vi "MSScript_Transform_BooleanArray.vi"(8 "MinSize":u8=1, 9 "MaxSize":u8=1, 11 "Check_Str":string) -> (2 "Value Error?":bool, 3 "Value Output":bool[](array[boolean]))   [LabVIEW 2018, in "MSScript.lvclass"]
uses:
  MSScript.lvclass
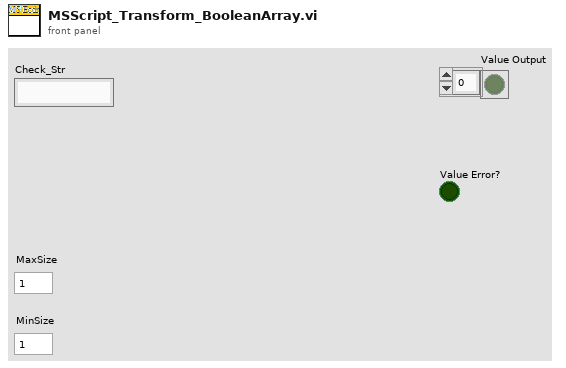
[diagram p1: front panel]
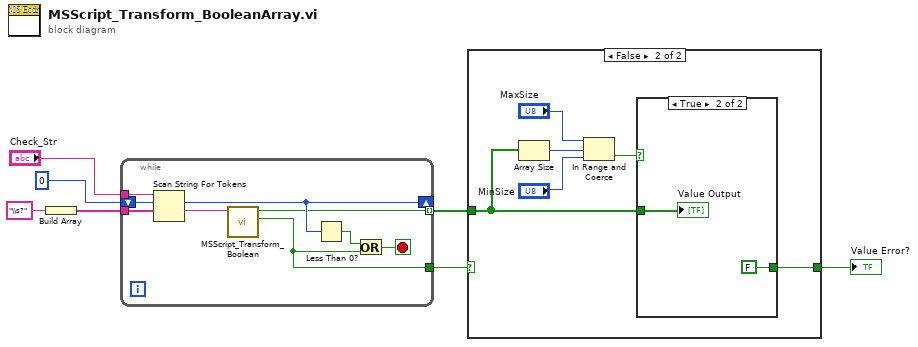
[diagram p0: block diagram]
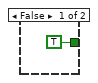
[diagram p3: hidden frame]
diagram:
  n1 = Build Array("\\s?" ("regular expression")) -> (w5:string[])
  n2 = while {
    tunnel: "Check_Str" -> [w16]
    tunnel: w5 -> [w11]
    shift-right: [w14] -> _
    shift-left: 0 ("offset") -> [w15]
    tunnel: [w9] -> w4
    tunnel: [w10] -> w3 mode=indexing
    stop <- w12 stop-if-true
    n3 = Scan String For Tokens(7:w11, 8:w15, 9:w16) -> (1:w8:string, 2:w14:i32)  [unwired: 3 in, 2 out]
    n4 = call "MSScript_Transform_Boolean.vi"("Check_Str"=w8) -> ("Value Error?"=w9:bool, "Value Output"=w10:bool)  [unwired: 9 in]
    n5 = Less Than 0?(x=w14) -> (x < 0?=w13:bool)
    n6 = Or(x=w13, y=w9) -> (x .or. y?=w12:bool)
  }
  n7 = case shown="False" w4 {
    selector: w4 -> [w17 _]
    tunnel: w3 -> [_ w22]
    tunnel: [w17 w20] -> w2
    frame True {
    }
    frame False {
      n8 = Array Size(array=w22) -> (size(s)=w23:i32)
      n9 = In Range and Coerce(upper limit="MaxSize", x=w23, lower limit="MinSize") -> (In Range?=w21:bool)  [unwired: 1 out]
      n10 = case shown="True" w21 {
        tunnel: w22 -> [_ w25]
        tunnel: [TRUE FALSE] -> w20
        frame False {
        }
        frame True {
          "Value Output" <- w25
        }
      }
    }
  }
  "Value Error?" <- w2
